vi "ContCompTime2Feed.vi"(10 "Refresh ratio per reactor":dbl, 11 "Param 1":dbl) -> (3 "Time [ms]":dbl)   [LabVIEW 2018, in "ContinousLoop.lvlib"]
uses:
  ContinousLoop.lvlib
  Arduino/VIs/Arduino.lvlib
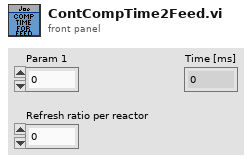
[diagram p1: front panel]
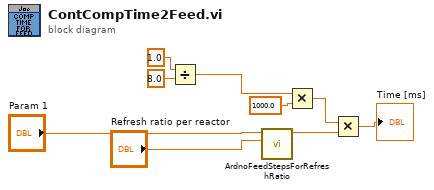
[diagram p0: block diagram]
diagram:
  n1 = Divide(x=1.0, y=8.0) -> (x/y=w5:dbl)
  n2 = call "ArdnoFeedStepsForRefreshRatio.vi"("ReactorRefreshRatio"="Refresh ratio per reactor", "Desired Refresh Ratio"="Param 1") -> ("Feed steps for the\n desired refresh ratio"=w8:dbl)  [unwired: 9 in]
  n3 = Multiply(x=w5, y=1000.0) -> (x*y=w7:dbl)
  n4 = Multiply(x=w7, y=w8) -> (x*y=→"Time [ms]":dbl)
